vi "SoundLoader.vi"() -> ()   [LabVIEW 2019, in "Initializers.lvlib"]
uses:
  Initializers.lvlib
  <vilib>/sound2/lvsound2.llb/Sound File Read Open.vi
  <vilib>/sound2/lvsound2.llb/Sound File Read (DBL).vi
panel:
  out "Array":i32[](array[numeric])
  out "Waveform Graph":i16[][](graph)
  out "error out 2":errorcluster
  in  "error out":errorcluster
  in  "Target Path":path=path "C:/Users/FreshBob/Dropbox/VIs/myRIO_GameConsole/Data/snake.sounds"
  in  "Paths":path[](array[path])=[path "C:/Users/FreshBob/Dropbox/VIs/myRIO_GameConsole/Data/Sounds/click.wav", path "C:/Users/FreshBob/Dropbox/VIs/myRIO_GameConsole/Data/Sounds/bling.wav", path "C:/Users/FreshBob/Dropbox/VIs/myRIO_GameConsole/Data/Sounds/boing.wav", path "C:/Users/FreshBob/Dropbox/VIs/myRIO_GameConsole/Data/Sounds/kick.wav", path "C:/Users/FreshBob/Dropbox/VIs/myRIO_GameConsole/Data/Sounds/youwin.wav"]
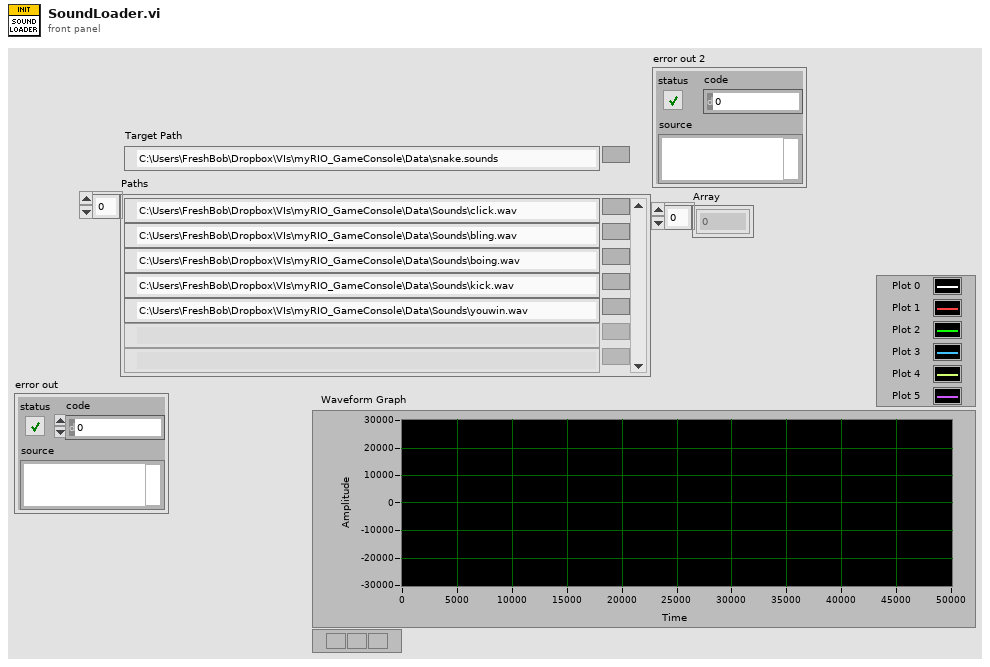
[diagram p1: front panel]
types:
  T1 = enum16{"open", "replace", "create", "open or create", "replace or create", "replace or create with confirmation"}
  T2 = typedef "Sound File Refnum.ctl" = refnum<file>
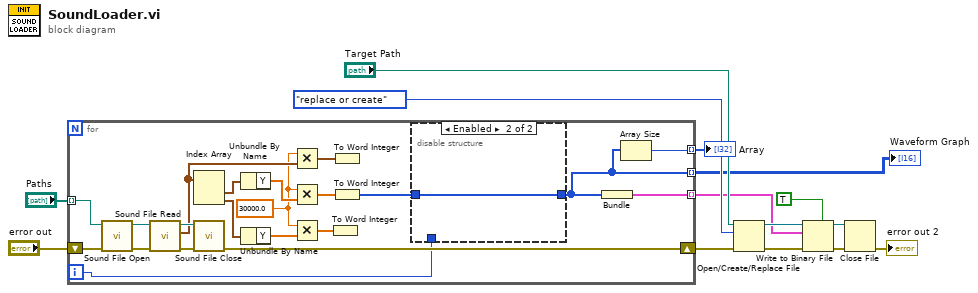
[diagram p0: block diagram]
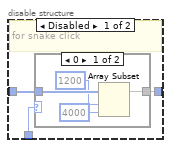
[diagram p2: hidden frame]
diagram:
  n1 = for {
    shift-right: [w31] -> w7
    shift-left: "error out" -> [w30]
    tunnel: "Paths" -> [w29] mode=indexing
    tunnel: [w19] -> w3 mode=indexing
    tunnel: [w16] -> w2 mode=indexing
    tunnel: [w17] -> w1 mode=indexing
    i -> [w15]
    w20 = 30000.0 ("x")
    n2 = call-poly <vilib>:"Sound File Open.vi"("error in (no error)"=w30, "path"=w29) -> ("error out"=w34:errorcluster, "sound file refnum"=w35:T2)  [unwired: 8 in]
    n3 = call-poly <vilib>:"Sound File Read.vi"("error in (no error)"=w34, "sound file refnum"=w35) -> ("error out"=w32:errorcluster, "data"=w24:waveform(dbl)[], "sound file refnum out"=w33:T2)  [unwired: 5 in, 2 out]
    n4 = Index Array(array=w24) -> (element #1=w28:waveform(dbl), element #2=w27:waveform(dbl))  [unwired: 2 in]
    n5 = call <vilib>:"Sound File Close.vi"("error in (no error)"=w32, "sound file refnum"=w33) -> ("error out"=w31:errorcluster)  [unwired: 9 in]
    n6 = Unbundle By Name(w28) -> ("Y"=w25:dbl[])
    n7 = Unbundle By Name(w27) -> ("Y"=w26:dbl[])
    n8 = Multiply(x=w20, y=w24) -> (x*y=w21:waveform(dbl)[])
    n9 = Multiply(x=w20, y=w25) -> (x*y=w23:dbl[])
    n10 = Multiply(x=w20, y=w26) -> (x*y=w22:dbl[])
    n11 = To Word Integer(number=w22) -> ()  [unwired: 1 out]
    n12 = To Word Integer(number=w21) -> ()  [unwired: 1 out]
    n13 = To Word Integer(number=w23) -> (16bit integer=w18:i16[])
    n14 = disable-structure shown="Enabled" {
      disable-tunnel: w18 -> [w38 w44]
      disable-tunnel: [w37 w44] -> w16
      disable-tunnel: w15 -> [w36 _]
      frame Disabled {
        # "for snake click"
        n15 = case shown="0" w36 {
          tunnel: w38 -> [w42 w43]
          tunnel: [w41 w43] -> w37
          frame 0 {
            n16 = Array Subset(array=w42, index=1200, length=4000) -> (w41:i16[])
          }
          frame 1, Default {
          }
        }
      }
      frame Enabled {
      }
    }
    n17 = Bundle(w16) -> (w19:cluster{i16[]})  [unwired: 1 in]
    n18 = Array Size(array=w16) -> (size(s)=w17:i32)
  }
  "Waveform Graph" <- w2
  "Array" <- w1
  n19 = Open/Create/Replace File(file path (use dialog)="Target Path", error in=w7, operation (0:open)=T1."replace or create") -> (refnum out=w14:refnum<file>, error out=w13:errorcluster)  [unwired: 3 in, 1 out]
  n20 = Write to Binary File(file (use dialog)=w14, data=w3, error in=w13, 5:TRUE ("prepend array or string size? (T)")) -> (refnum out=w12:refnum<file>, error out=w11:errorcluster)  [unwired: 2 in, 1 out]
  n21 = Close File(refnum=w12, error in=w11) -> (error out=→"error out 2":errorcluster)  [unwired: 1 out]
